vi "generateTestData.vi"() -> ()   [LabVIEW 2016]
panel:
  out "Aeration [%]":dbl
  out "CO2 [10000ppm]":dbl
  out "Flow":dbl
  out "Turbidity":dbl
  out "Temperature":dbl
  out "Substrate dosing":bool
  out "Redox":dbl
  out "Recycle":bool
  out "pH":dbl
  out "Oxygen":dbl
  out "Overflow":bool
  out "Mixing [%]":dbl
  out "Mixer":bool
  out "Feed":bool
  out "CO2 [3000ppm]":dbl
  out "Aeration":bool
  out "Level":dbl
  in  "Stop Button":bool
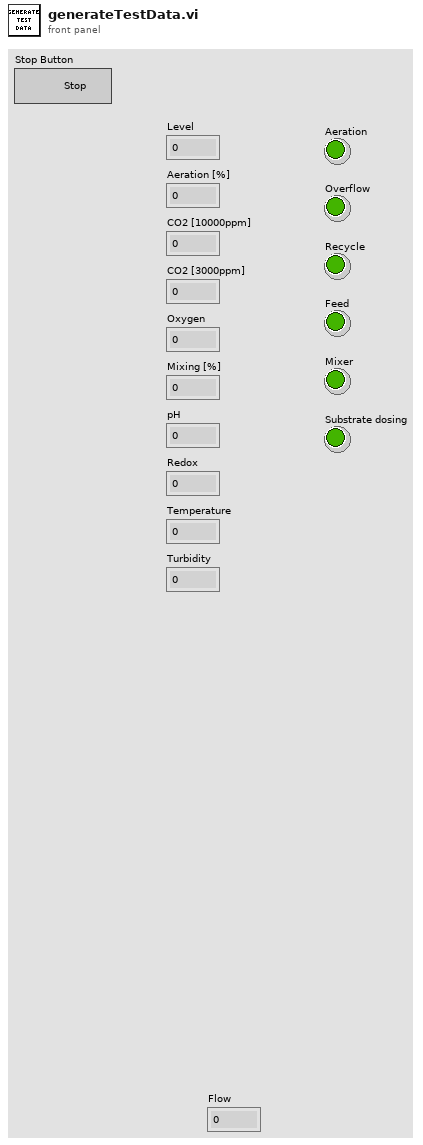
[diagram p1: front panel]
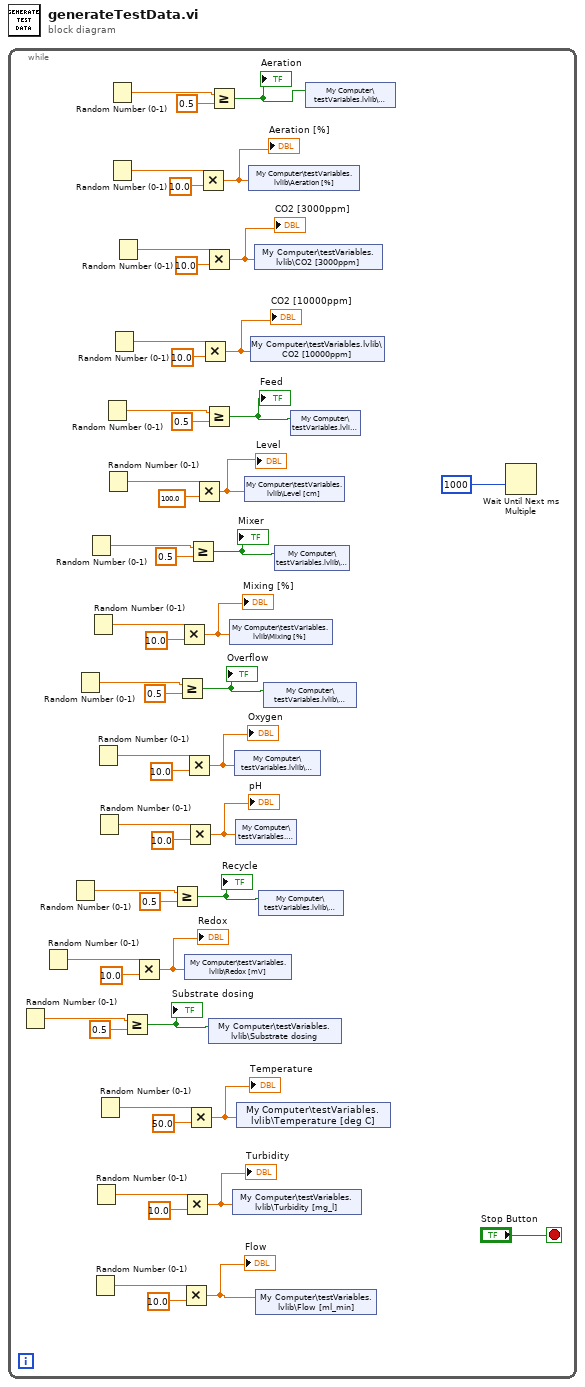
[diagram p0: block diagram]
diagram:
  n1 = while {
    stop <- "Stop Button" stop-if-true
    n2 = Random Number (0-1)() -> (number: 0 to 1=w18:dbl)
    n3 = Random Number (0-1)() -> (number: 0 to 1=w21:dbl)
    n4 = Random Number (0-1)() -> (number: 0 to 1=w24:dbl)
    n5 = Random Number (0-1)() -> (number: 0 to 1=w33:dbl)
    n6 = Random Number (0-1)() -> (number: 0 to 1=w39:dbl)
    n7 = Random Number (0-1)() -> (number: 0 to 1=w36:dbl)
    n8 = Random Number (0-1)() -> (number: 0 to 1=w9:dbl)
    n9 = Random Number (0-1)() -> (number: 0 to 1=w12:dbl)
    n10 = Random Number (0-1)() -> (number: 0 to 1=w30:dbl)
    n11 = Random Number (0-1)() -> (number: 0 to 1=w27:dbl)
    n12 = Random Number (0-1)() -> (number: 0 to 1=w15:dbl)
    n13 = Random Number (0-1)() -> (number: 0 to 1=w42:dbl)
    n14 = Random Number (0-1)() -> (number: 0 to 1=w51:dbl)
    n15 = Random Number (0-1)() -> (number: 0 to 1=w48:dbl)
    n16 = Random Number (0-1)() -> (number: 0 to 1=w3:dbl)
    n17 = Random Number (0-1)() -> (number: 0 to 1=w6:dbl)
    n18 = Random Number (0-1)() -> (number: 0 to 1=w45:dbl)
    n19 = Greater Or Equal?(x=w18, y=0.5) -> (x >= y?=w16:bool)
    "Substrate dosing" <- w16
    n20 = Multiply(x=w21, y=10.0) -> (x*y=w19:dbl)
    "Redox" <- w19
    n21 = Greater Or Equal?(x=w24, y=0.5) -> (x >= y?=w22:bool)
    "Recycle" <- w22
    n22 = Greater Or Equal?(x=w33, y=0.5) -> (x >= y?=w31:bool)
    "Overflow" <- w31
    n23 = Multiply(x=w36, y=10.0) -> (x*y=w34:dbl)
    "Mixing [%]" <- w34
    n24 = Multiply(x=w9, y=10.0) -> (x*y=w7:dbl)
    "Flow" <- w7
    n25 = Multiply(x=w12, y=10.0) -> (x*y=w10:dbl)
    "Turbidity" <- w10
    n26 = Multiply(x=w30, y=10.0) -> (x*y=w28:dbl)
    "Oxygen" <- w28
    n27 = Multiply(x=w27, y=10.0) -> (x*y=w25:dbl)
    "pH" <- w25
    n28 = shared-variable "My Computer\\testVariables.lvlib\\Redox [mV]"(w19) -> ()  [unwired: 1 in, 1 out]
    n29 = Multiply(x=w15, y=50.0) -> (x*y=w13:dbl)
    "Temperature" <- w13
    n30 = Greater Or Equal?(x=w39, y=0.5) -> (x >= y?=w37:bool)
    "Mixer" <- w37
    n31 = Multiply(x=w51, y=100.0) -> (x*y=w49:dbl)
    "Level" <- w49
    n32 = Multiply(x=w3, y=10.0) -> (x*y=w1:dbl)
    "Aeration [%]" <- w1
    n33 = Multiply(x=w6, y=10.0) -> (x*y=w4:dbl)
    "CO2 [10000ppm]" <- w4
    n34 = Multiply(x=w45, y=10.0) -> (x*y=w43:dbl)
    "CO2 [3000ppm]" <- w43
    n35 = Greater Or Equal?(x=w42, y=0.5) -> (x >= y?=w40:bool)
    "Feed" <- w40
    n36 = Greater Or Equal?(x=w48, y=0.5) -> (x >= y?=w46:bool)
    "Aeration" <- w46
    n37 = shared-variable "My Computer\\testVariables.lvlib\\Substrate dosing"(w16) -> ()  [unwired: 1 in, 1 out]
    n38 = shared-variable "My Computer\\testVariables.lvlib\\Mixing [%]"(w34) -> ()  [unwired: 1 in, 1 out]
    n39 = shared-variable "My Computer\\testVariables.lvlib\\Turbidity [mg_l]"(w10) -> ()  [unwired: 1 in, 1 out]
    n40 = shared-variable "My Computer\\testVariables.lvlib\\Oxygen"(w28) -> ()  [unwired: 1 in, 1 out]
    n41 = shared-variable "My Computer\\testVariables.lvlib\\pH"(w25) -> ()  [unwired: 1 in, 1 out]
    n42 = shared-variable "My Computer\\testVariables.lvlib\\Temperature [deg C]"(w13) -> ()  [unwired: 1 in, 1 out]
    n43 = shared-variable "My Computer\\testVariables.lvlib\\Level [cm]"(w49) -> ()  [unwired: 1 in, 1 out]
    n44 = shared-variable "My Computer\\testVariables.lvlib\\Aeration [%]"(w1) -> ()  [unwired: 1 in, 1 out]
    n45 = shared-variable "My Computer\\testVariables.lvlib\\CO2 [10000ppm]"(w4) -> ()  [unwired: 1 in, 1 out]
    n46 = shared-variable "My Computer\\testVariables.lvlib\\CO2 [3000ppm]"(w43) -> ()  [unwired: 1 in, 1 out]
    n47 = shared-variable "My Computer\\testVariables.lvlib\\Flow [ml_min]"(w7) -> ()  [unwired: 1 in, 1 out]
    n48 = shared-variable "My Computer\\testVariables.lvlib\\Recycle"(w22) -> ()  [unwired: 1 in, 1 out]
    n49 = shared-variable "My Computer\\testVariables.lvlib\\Overflow"(w31) -> ()  [unwired: 1 in, 1 out]
    n50 = shared-variable "My Computer\\testVariables.lvlib\\Mixer"(w37) -> ()  [unwired: 1 in, 1 out]
    n51 = shared-variable "My Computer\\testVariables.lvlib\\Feed"(w40) -> ()  [unwired: 1 in, 1 out]
    n52 = shared-variable "My Computer\\testVariables.lvlib\\Aeration"(w46) -> ()  [unwired: 1 in, 1 out]
    n53 = Wait Until Next ms Multiple(millisecond multiple=u32 1000) -> ()  [unwired: 1 out]
  }
